vi "normalize_to_TF.vi"(8 "TF phase":dbl[](array[numeric]), 9 "TF mag":dbl[](array[numeric]), 11 "signal (can be complex)":cdb[](array[numeric])) -> (3 "signal normalized to TF (can be complex)":cdb[](array[numeric]))   [LabVIEW 2021]
panel:
  out "size(s) 2":i32
  out "size(s)":i32
  out "TF complex":cdb[](array[numeric])
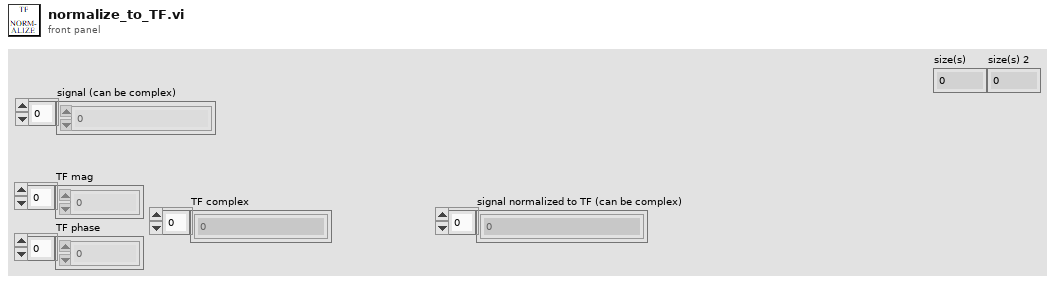
[diagram p1: front panel]
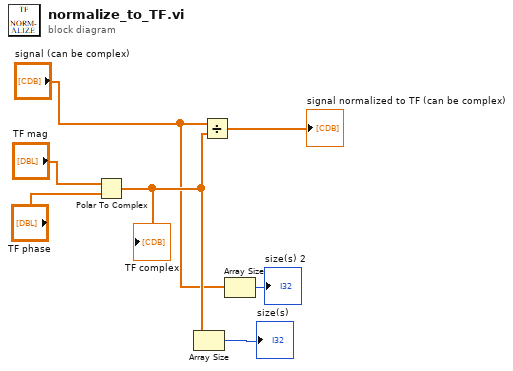
[diagram p0: block diagram]
diagram:
  n1 = Polar To Complex(1:"TF phase", 2:"TF mag") -> (0:w4:cdb[])
  "TF complex" <- w4
  n2 = Array Size(array=w4) -> (size(s)=→"size(s)":i32)
  n3 = Divide(x="signal (can be complex)", y=w4) -> (x/y=→"signal normalized to TF (can be complex)":cdb[])
  n4 = Array Size(array="signal (can be complex)") -> (size(s)=→"size(s) 2":i32)
